vi "gantry_rot_run.vi"(8 "VISA resource name":refnum<visa-resource-name>="COM7", 10 "dir":dbl=1.0, 11 "desired motor speed (T/2) [us]":dbl=350.0) -> (0 "VISA resource name out":refnum<visa-resource-name>, 3 "Target speed input to Arduino":dbl=35.0)   [LabVIEW 2021]
panel:
  in  "microcrontroller dt [us]":dbl=10.0 format="%#_13g"
  in  "Starting T/2 Arduino":dbl=500.0
  in  "Period update extension":dbl=200.0
  in  "Ramping delta":dbl=8.0
  out "read buffer":string
  out "resulting string":string="R35 5 8 200 400 1"
  in  "ramping rate":dbl=5.0
  # "Note: to change motor ramping speed, best to change \"Starting T/2 Arduino\""
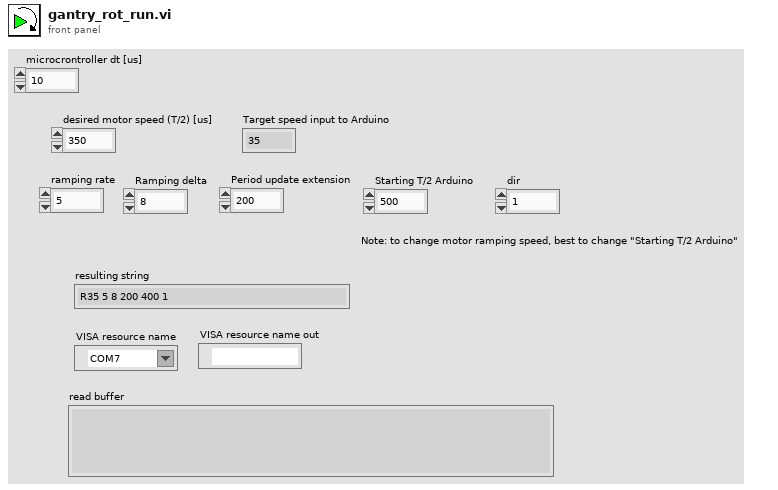
[diagram p1: front panel]
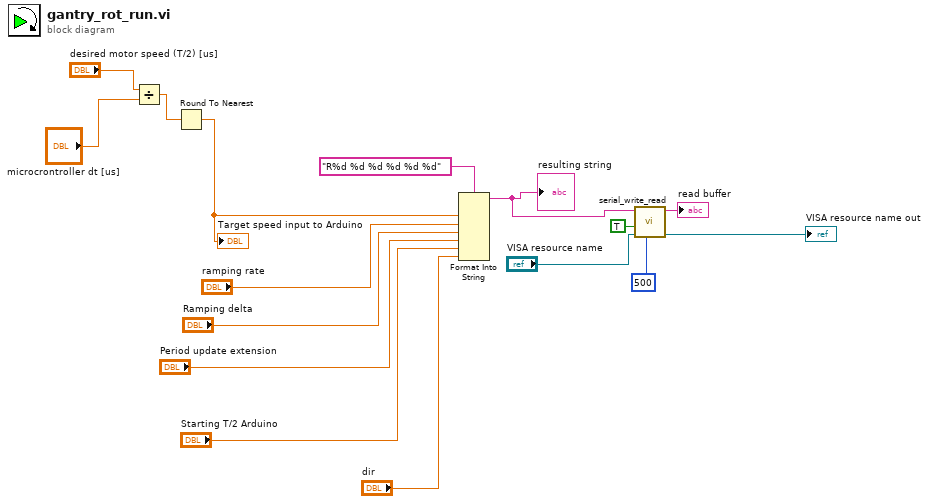
[diagram p0: block diagram]
diagram:
  n1 = Divide(x="desired motor speed (T/2) [us]", y="microcrontroller dt [us]") -> (x/y=w11:dbl)
  n2 = Round To Nearest(number=w11) -> (nearest integer value=w10:dbl)
  "Target speed input to Arduino" <- w10
  n3 = Format Into String(format string="R%d %d %d %d %d %d", w10, "ramping rate", "Ramping delta", "Period update extension", "Starting T/2 Arduino", "dir") -> (resulting string=w14:string)  [unwired: 2 in, 1 out]
  "resulting string" <- w14
  n4 = call "serial_write_read.vi"("read byte count"=u32 500, "VISA resource name"="VISA resource name", "Clear buffer"=TRUE, "write buffer"=w14) -> ("VISA resource name out"=→"VISA resource name out":refnum<visa-resource-name>, "read buffer"=→"read buffer":string)  [unwired: 6 in]
